vi "color in range.vi"(3 "variance":u8=20, 4 "target color":u32(colorbox), 5 "Color":u32(colorbox)) -> (1 "in range?":bool)   [LabVIEW 2009]
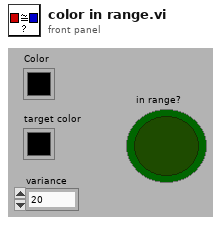
[diagram p1: front panel]
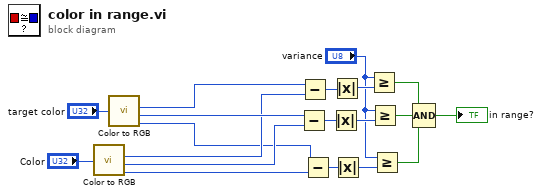
[diagram p0: block diagram]
diagram:
  n1 = call <vilib>:"Color to RGB.vi"("Color"="Color") -> ("R"=w15:u8, "G"=w14:u8, "B"=w13:u8)  [unwired: 1 out]
  n2 = call <vilib>:"Color to RGB.vi"("Color"="target color") -> ("R"=w17:u8, "G"=w16:u8, "B"=w9:u8)  [unwired: 1 out]
  n3 = Subtract(x=w16, y=w14) -> (x-y=w11:i16)
  n4 = Subtract(x=w17, y=w15) -> (x-y=w12:i16)
  n5 = Subtract(x=w9, y=w13) -> (x-y=w10:i16)
  n6 = Absolute Value(x=w11) -> (abs(x)=w8:i16)
  n7 = Absolute Value(x=w12) -> (abs(x)=w6:i16)
  n8 = Absolute Value(x=w10) -> (abs(x)=w7:i16)
  n9 = Greater Or Equal?(x="variance", y=w6) -> (x >= y?=w4:bool)
  n10 = Greater Or Equal?(x="variance", y=w8) -> (x >= y?=w3:bool)
  n11 = Greater Or Equal?(x="variance", y=w7) -> (x >= y?=w2:bool)
  n12 = Compound Arithmetic op=AND(w4, w3, w2) -> (→"in range?":bool)
